vi "Start If All Ready.vi"(8 "error in (no error)":errorcluster, 11 "Log Manager Module in":refnum<class "Log Manager Module.lvclass">) -> (0 "error out":errorcluster, 3 "Log Manager Module out":refnum<class "Log Manager Module.lvclass">)   [LabVIEW 2020, in "VolatusData.lvlib" / "Log Manager Module.lvclass"]
uses:
  Log Manager Module.lvclass
  C:/dev/lv20CE/relink/lv-volatus/Volatus/Module/Module.lvclass
  Log Manager Module.lvclass/Log Manager Module.ctl
  Logger State.ctl
  Logging State.ctl
  Volatus/Module/Module.lvclass/Module.ctl
  Volatus/MessageQ/MessageQ.lvclass/MessageQ.ctl
  Volatus/Module/Module.lvclass
  VolatusData.lvlib
  Volatus/MessageQ/MessageQ.lvclass
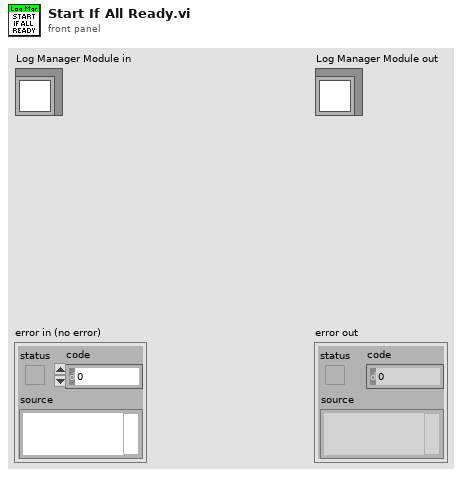
[diagram p1: front panel]
types:
  T1 = typedef "VolatusData.lvlib/Log Manager Module.lvclass/Logger.ctl" = cluster{"ID":string, "MsgQ":refnum<class "MessageQ.lvclass">, "State":T2}
  T2 = typedef "VolatusData.lvlib/Logger State.ctl" = enum16{"Unknown", "Idle", "Preparing", "Ready", "Logging", "Stopping"}
  T3 = typedef "VolatusData.lvlib/Logging State.ctl" = enum16{"Idle", "Starting", "Logging", "Stopping"}
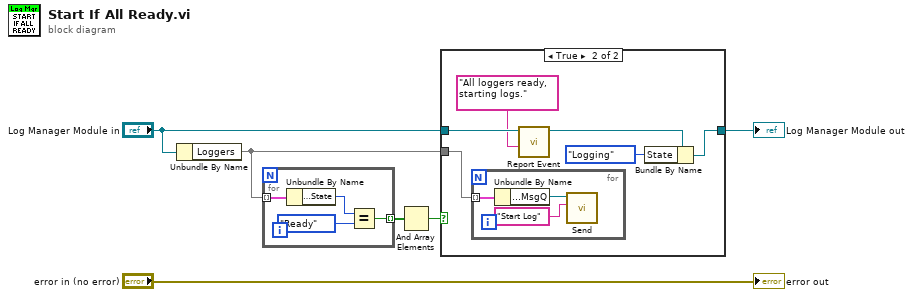
[diagram p0: block diagram]
diagram:
  n1 = Unbundle By Name("Log Manager Module in") -> ("Loggers"=w4:map{string, T1})
  n2 = for {
    tunnel: w4 -> [w10] mode=indexing
    tunnel: [w7] -> w6 mode=indexing
    n3 = Unbundle By Name(w10) -> ("Logger.State"=w9:T2)
    n4 = Equal?(x=w9, y=Logger_State."Ready") -> (x = y?=w7:bool)
  }
  n5 = And Array Elements(Boolean array=w6) -> (logical AND=w5:bool)
  n6 = case shown="True" w5 {
    tunnel: w4 -> [_ w15]
    tunnel: "Log Manager Module in" -> [w11 w17]
    tunnel: [w11 w12] -> w1
    frame False {
    }
    frame True {
      n7 = for {
        tunnel: w15 -> [w20] mode=indexing
        n8 = Unbundle By Name(w20) -> ("Logger.MsgQ"=w19:refnum<class "MessageQ.lvclass">)
        n9 = call "Send.vi"("ID"="Start Log", "MessageQ in"=w19) -> ()  [unwired: 8 in, 2 out]
      }
      n10 = call "Report Event.vi"("Message"="All loggers ready, starting logs.", "Module in"=w17) -> ("Module out"=w14:refnum<class "Log Manager Module.lvclass">)  [unwired: 8 in, 1 out]
      n11 = Bundle By Name(cluster=w14, "State"=Logging_State."Logging") -> (w12:refnum<class "Log Manager Module.lvclass">)
    }
  }
  "Log Manager Module out" <- w1
  "error out" <- "error in (no error)"
